vi "Set waveform acquiring.vi"() -> ()   [LabVIEW 2020]
panel:
  in  "VISA resource name":refnum<visa-resource-name>
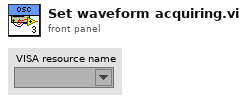
[diagram p1: front panel]
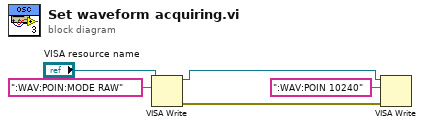
[diagram p0: block diagram]
diagram:
  n1 = VISA Write(VISA resource name="VISA resource name", write buffer=":WAV:POIN:MODE RAW") -> (VISA resource name out=w2:refnum<visa-resource-name>, error out=w3:errorcluster)  [unwired: 1 in, 1 out]
  n2 = VISA Write(VISA resource name=w2, write buffer=":WAV:POIN 10240", error in (no error)=w3) -> ()  [unwired: 3 out]
